vi "当前时间格式显示 (子VI).vi"() -> (3 "当前时间格式显示":string)   [LabVIEW 2016, in "数据传输系统.lvlib"]
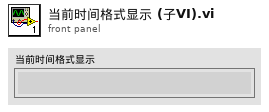
[diagram p1: front panel]
types:
  T1 = typedef "LVDateTimeRec.ctl" = cluster{"秒数的小数部分":dbl, "秒":i32, "分":i32, "时":i32, "日":i32, "月":i32, "年":i32, "天数（周）":i32, "天数（年）":i32, "DST":i32}
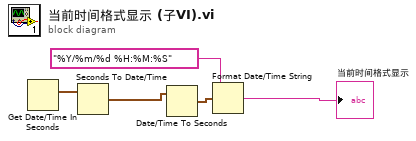
[diagram p0: block diagram]
diagram:
  n1 = Get Date/Time In Seconds() -> (seconds since 1Jan1904=w5:timestamp)
  n2 = Seconds To Date/Time(time stamp (now)=w5) -> (date time rec=w2:T1)  [unwired: 1 in]
  n3 = Date/Time To Seconds(2:w2) -> (0:w4:timestamp)  [unwired: 1 in]
  n4 = Format Date/Time String(time format string (%c)="%Y/%m/%d %H:%M:%S" ("时间格式字符串(%c)"), seconds (now)=w4) -> (date/time string=→"当前时间格式显示":string)  [unwired: 1 in]
